vi "XML - Create XML file.vi"(8 "error in (no error)":errorcluster, 11 "CD Wizard - Internal Data":T1) -> (0 "error out":errorcluster, 3 "XML file path":path)   [LabVIEW 2015]
doc: "Create the XML file and alter the content of the file, so that it fits for the generated custom device."
uses:
  TypDef/CD Wizard - Internal data.ctl
  TypDef/CD Wizard - Execution Mode.ctl
  TypDef/CD Wizard - Extra Page Name and GUID.ctl
  TypDef/Create XML-file - States.ctl
  Constants/Constants TypDef/XML File.ctl
  Constants/Constants TypDef/CD System Explorer lvlib.ctl
  TypDef/Target Type.ctl
  Constants/XML File.vi
  Constants/CD System Explorer lvlib.vi
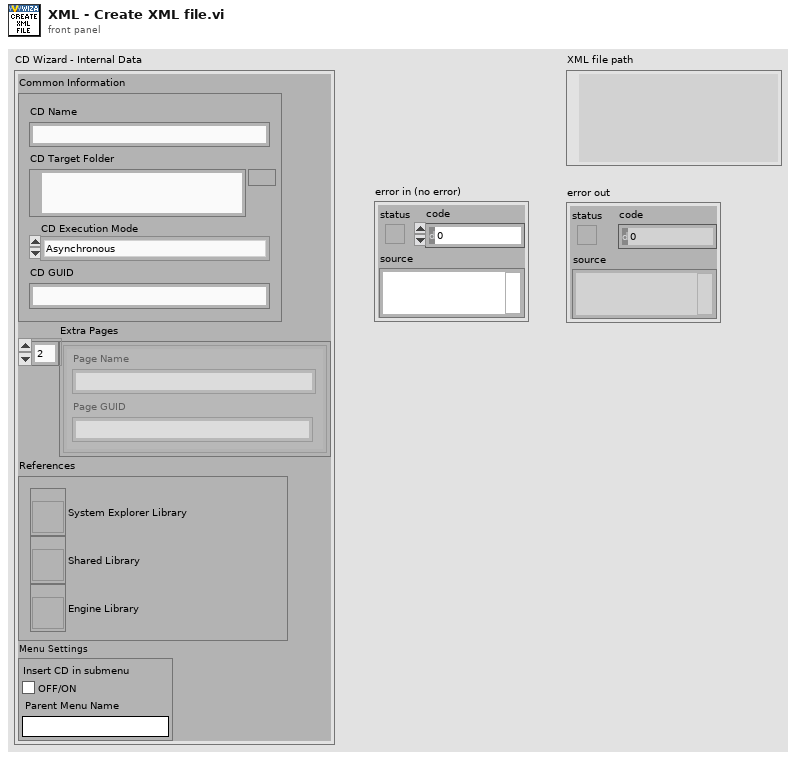
[diagram p1: front panel]
types:
  T1 = typedef "CD Wizard - Internal data.ctl" = cluster{"Common Information":cluster{"CD Name":string, "CD Target Folder":path, "CD Execution Mode":T2, "CD GUID":string}, "Extra Pages":T3[], "References":cluster{"System Explorer Library":refnum<vi>, "Shared Library":refnum<vi>, "Engine Library":refnum<vi>}, "Menu Settings":cluster{"Insert CD in submenu":bool, "Parent Menu Name":string}}
  T2 = typedef "CD Wizard - Execution Mode.ctl" = enum16{"Asynchronous", "Inline HW Interface", "Inline Model Interface", "Inline Timing and Sync", "Asynchronous Timing and Sync"}
  T3 = typedef "CD Wizard - Extra Page Name and GUID.ctl" = cluster{"Page Name":string, "Page GUID":string}
  T4 = typedef "Create XML-file - States.ctl" = enum16{"Initialize", "Copy XML template file", "Read XML file content", "Change CD -MenuName-", "Change CD -Name-", "Change CD -Type-", "Change CD -MainPageGUID-", "Change CD -InitVIPath-", "Change CD -WindowsCustomDeviceVIPath-", "Change CD -WindowsCustomDeviceVIRTPath-", "Change CD -PharlapCustomDeviceVIPath-", "Change CD -PharlapCustomDeviceVIRTPath-", "Change CD -VxWorksCustomDeviceVIPath-", "Change CD -VxWorksCustomDeviceVIRTPath-", "Change CD -LinuxARMCustomDeviceVIPath-", "Change CD -LinuxARMCustomDeviceVIRTPath-", "Change CD -Linuxx64CustomDeviceVIPath-", "Change CD -Linuxx64CustomDeviceVIRTPath-", "Change CD -MainPageVIPath-", "Change CD -ExtraPages-", "Write XML file content back", "Shutdown"}
  T5 = typedef "XML File.ctl" = enum16{"XMLTemplateFilePathAndName", "XMLTimingAndSyncFileName", "XMLCustomDeviceFileName"}
  T6 = typedef "CD System Explorer lvlib.ctl" = enum16{"LibraryFileName", "LibraryFolderName", "System Explorer.FolderName", "System Explorer.Dynamically Called.FolderName", "System Explorer.Dynamically Called.Extra Pages.FolderName", "System Explorer.Dynamically Called.Extra Pages.TemplatePathAndName", "System Explorer.Dynamically Called.Main Page.VIName", "System Explorer.Dynamically Called.Main Page.TemplatePathAndName", "System Explorer.Dynamically Called.Initialization VI.VIName", "System Explorer.Dynamically Called.Initialization VI.TemplatePathAndName", "System Explorer.SubVI.FolderName", "System Explorer.Types.FolderName"}
  T7 = typedef "Target Type.ctl" = enum16{"Windows", "VxWorks", "Pharlap", "Linux 32 ARM", "Linux x64"}
  T8 = enum16{"open", "replace", "create", "open or create", "replace or create", "replace or create with confirmation"}
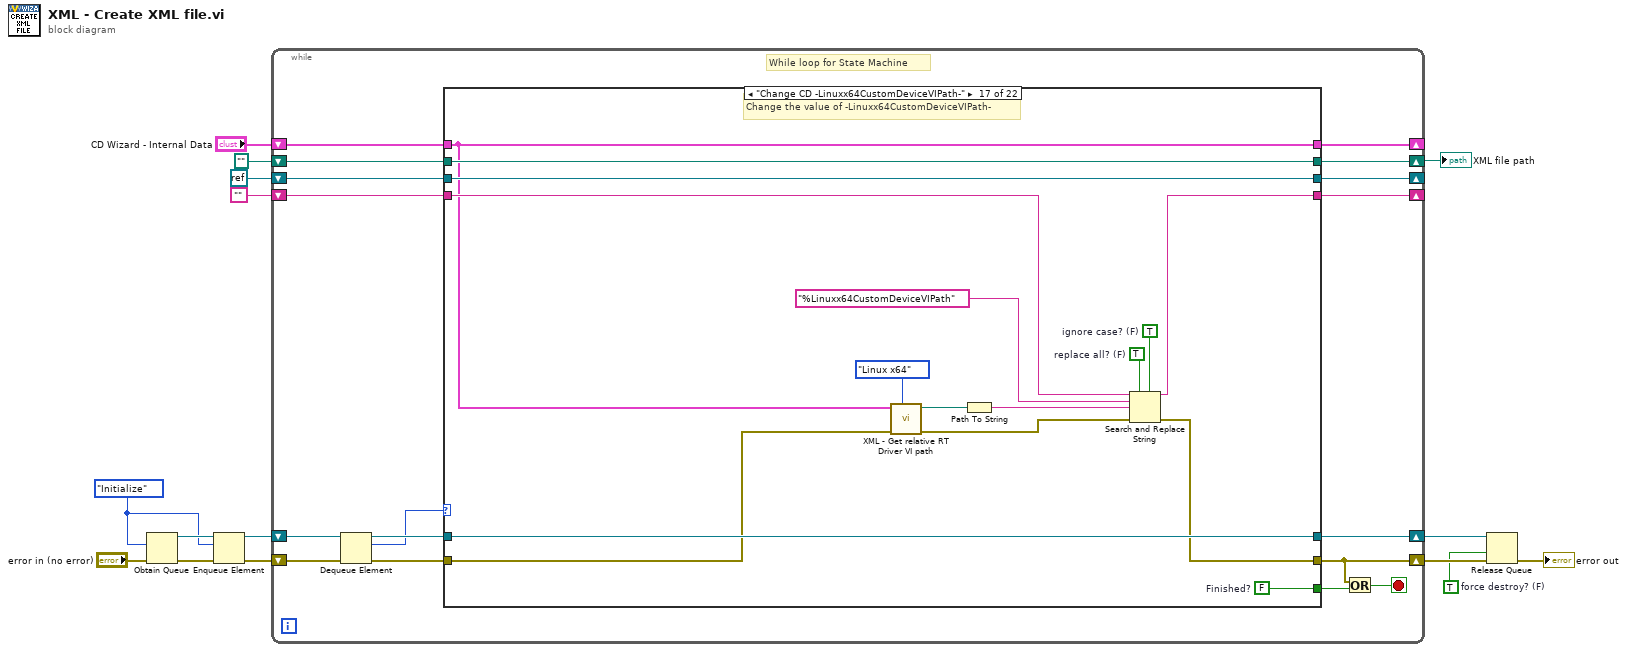
[diagram p0: block diagram]
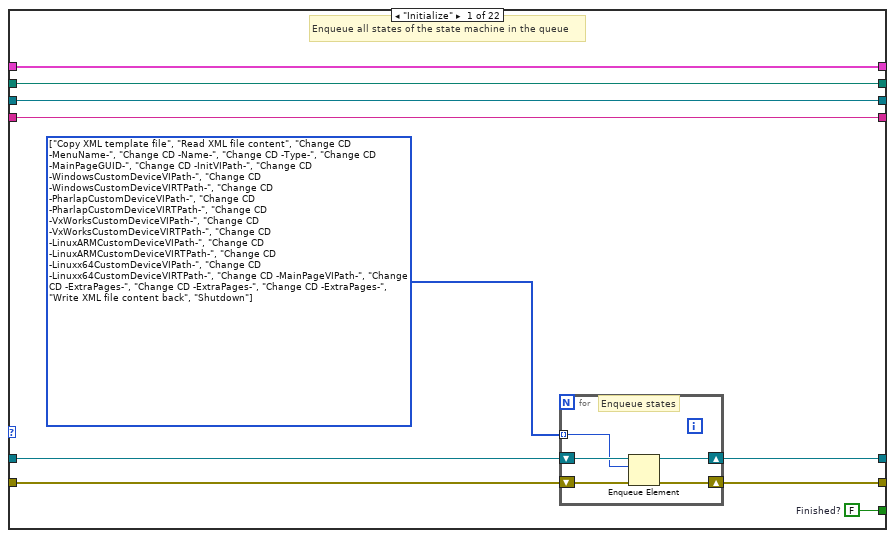
[diagram p2: hidden frame]
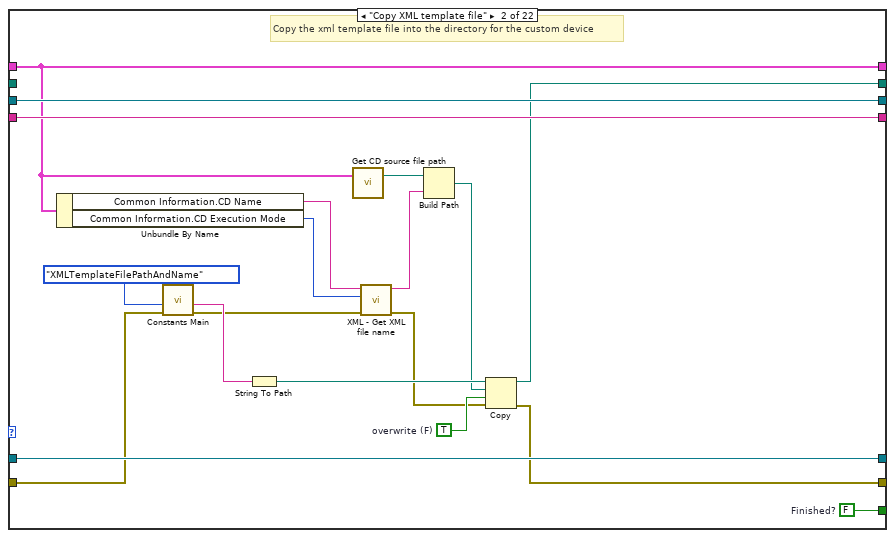
[diagram p3: hidden frame]
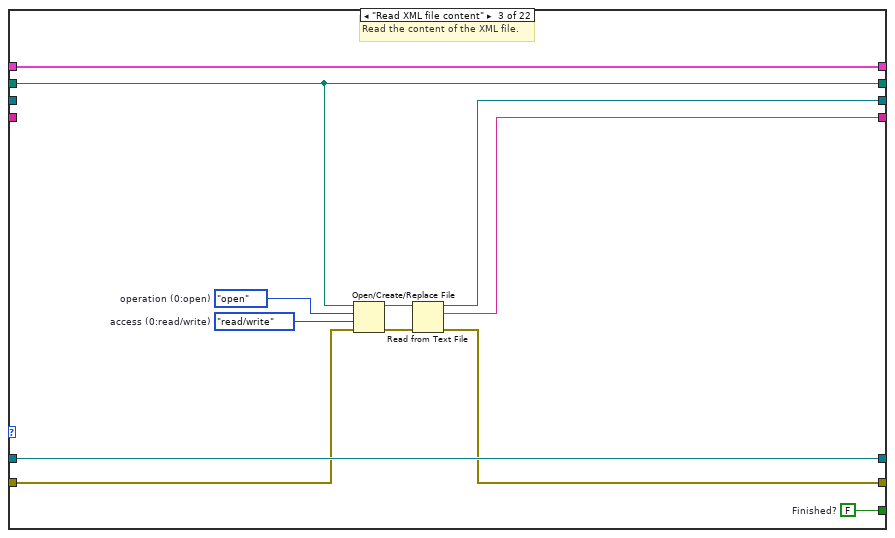
[diagram p4: hidden frame]
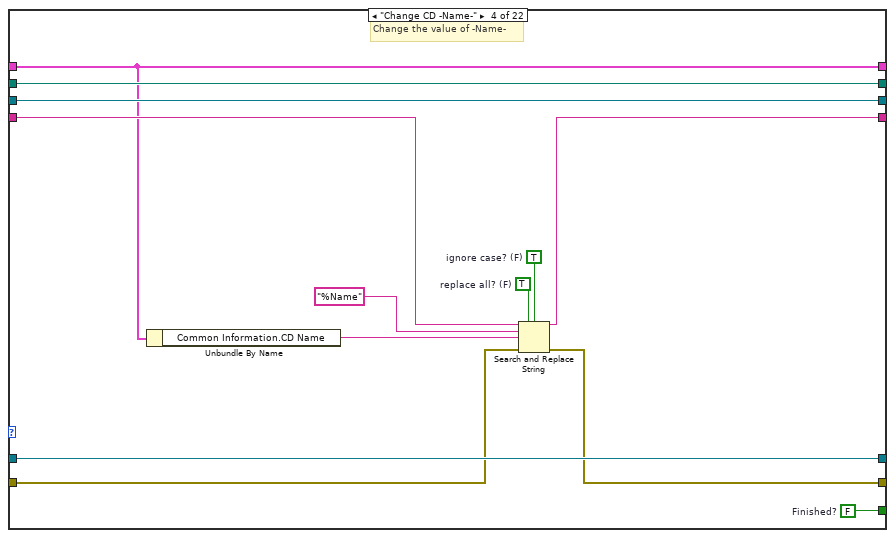
[diagram p5: hidden frame]
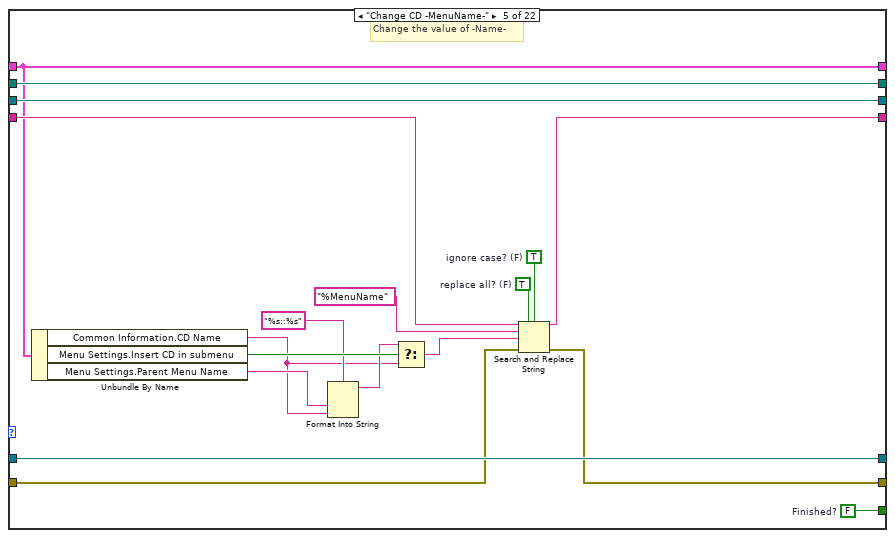
[diagram p6: hidden frame]
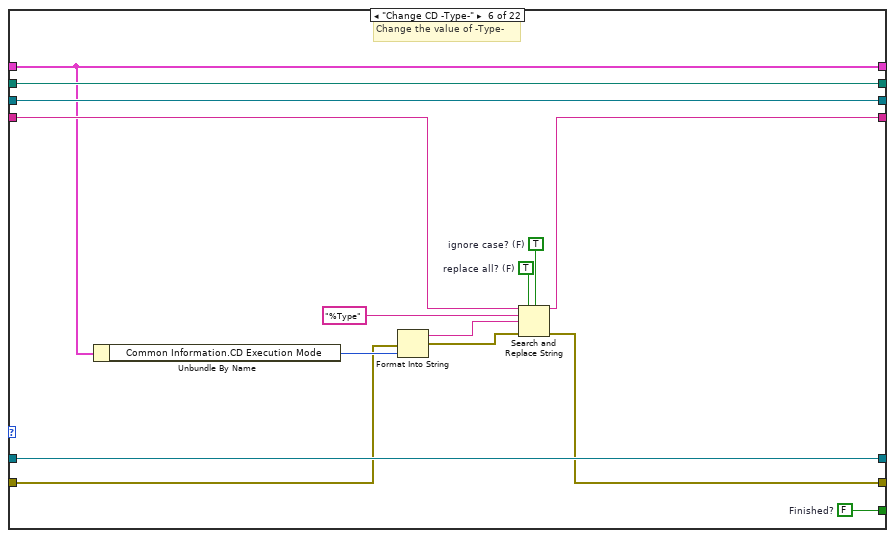
[diagram p7: hidden frame]
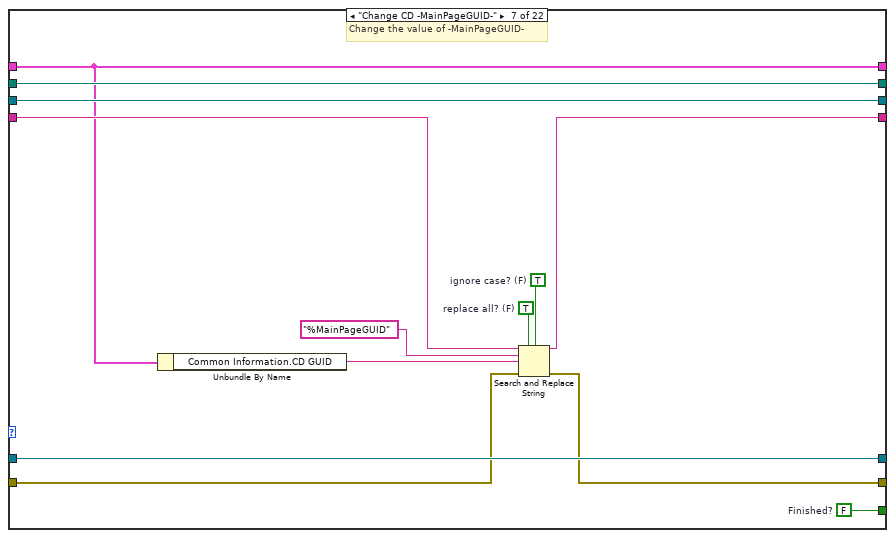
[diagram p8: hidden frame]
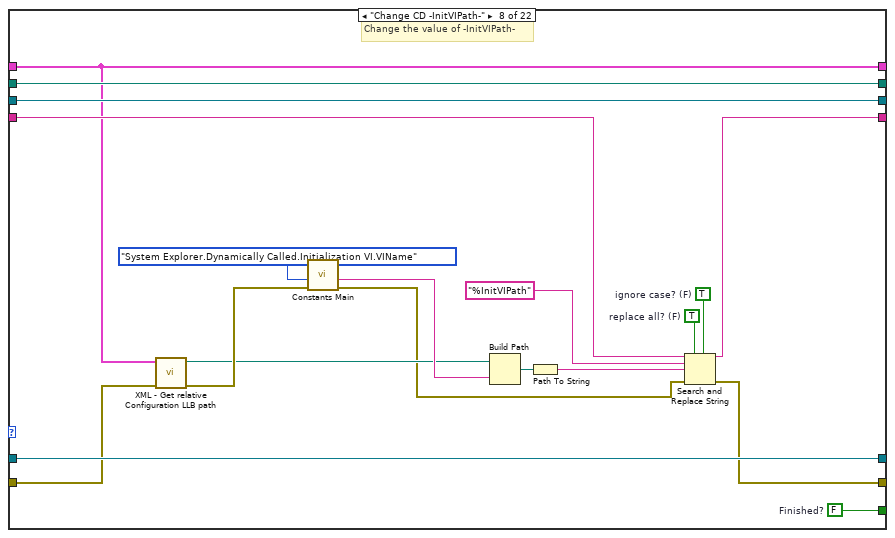
[diagram p9: hidden frame]
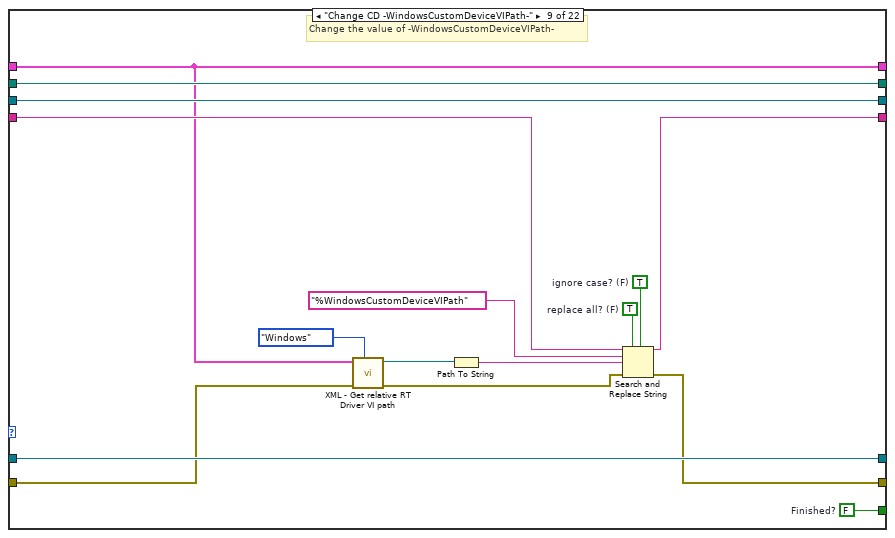
[diagram p10: hidden frame]
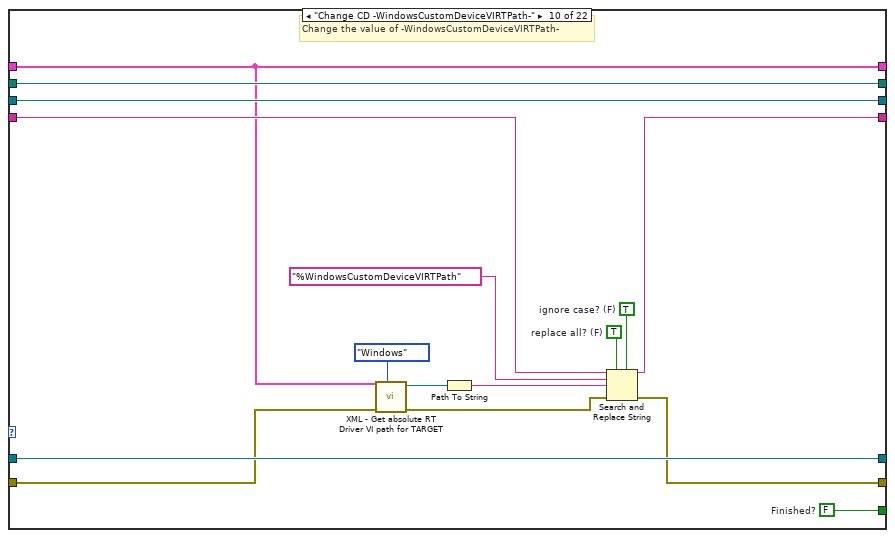
[diagram p11: hidden frame]
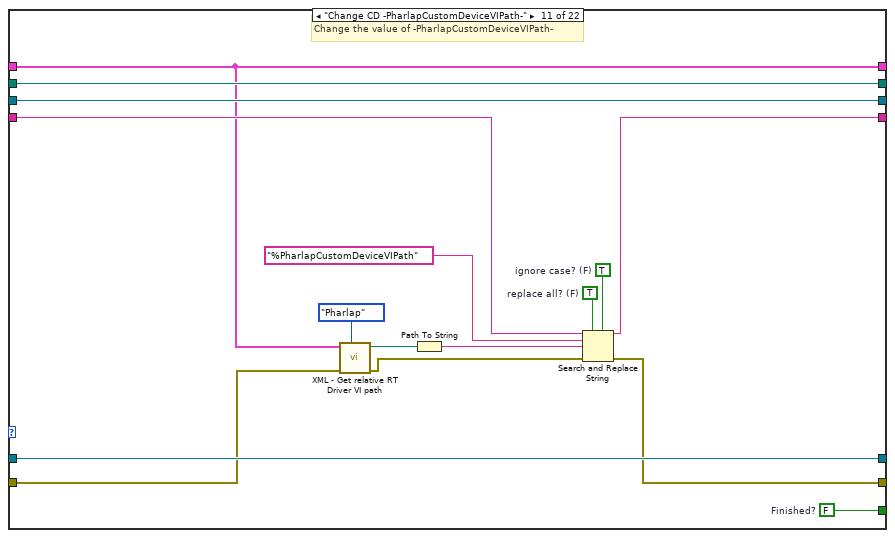
[diagram p12: hidden frame]
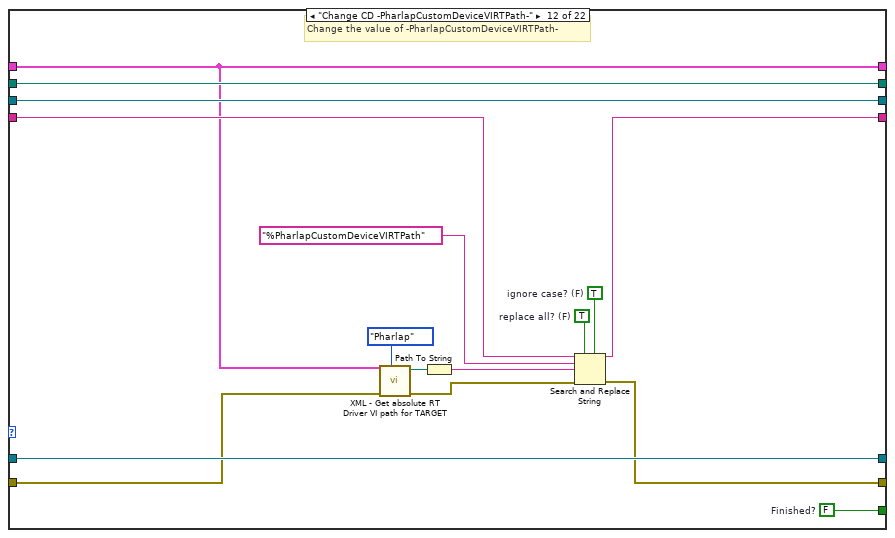
[diagram p13: hidden frame]
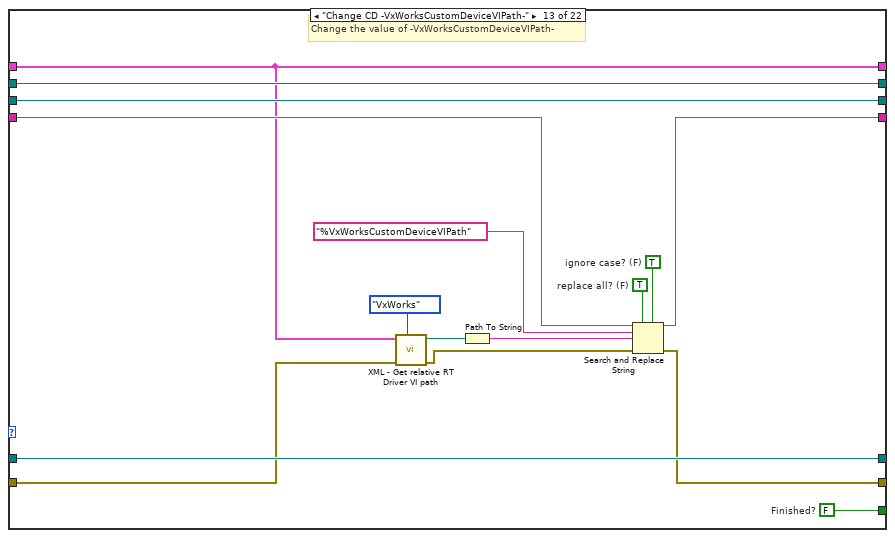
[diagram p14: hidden frame]
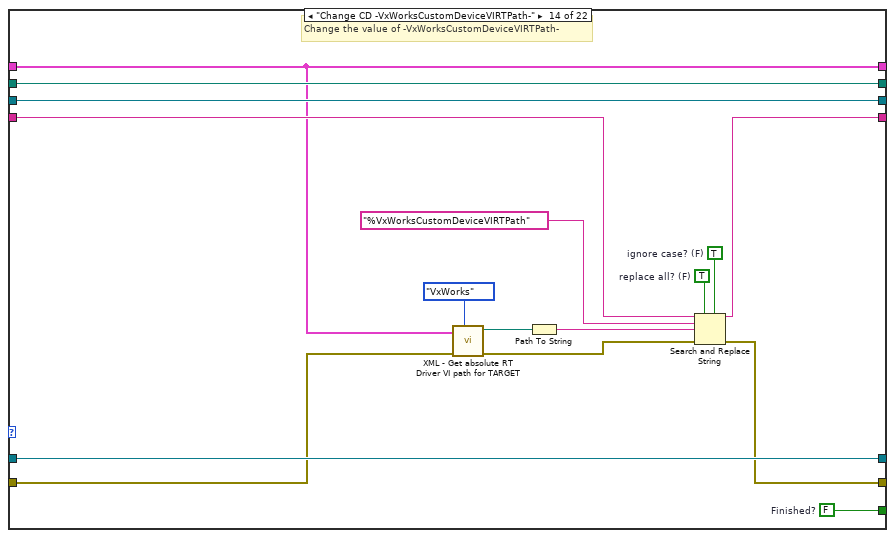
[diagram p15: hidden frame]
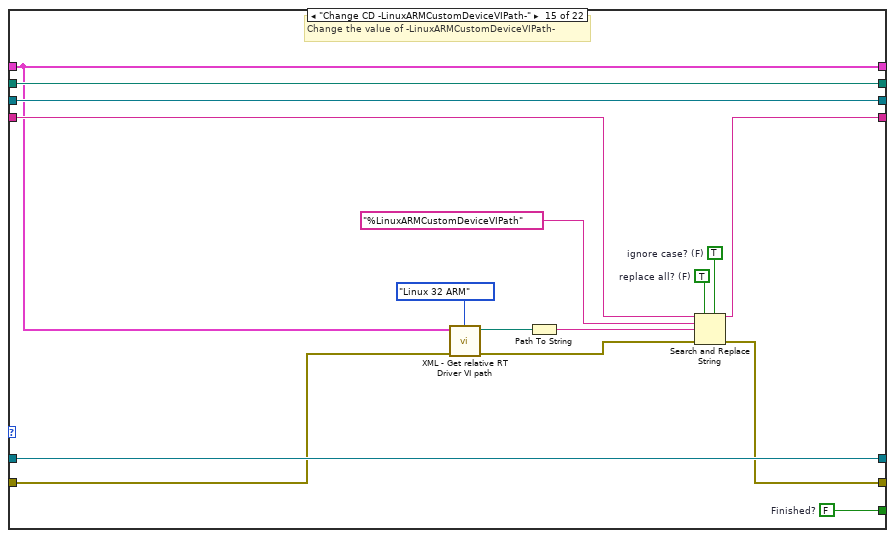
[diagram p16: hidden frame]
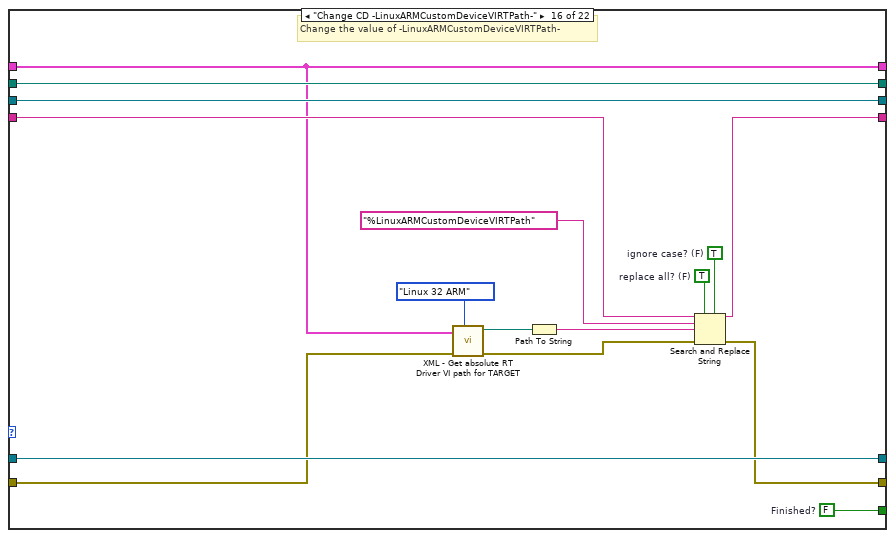
[diagram p17: hidden frame]
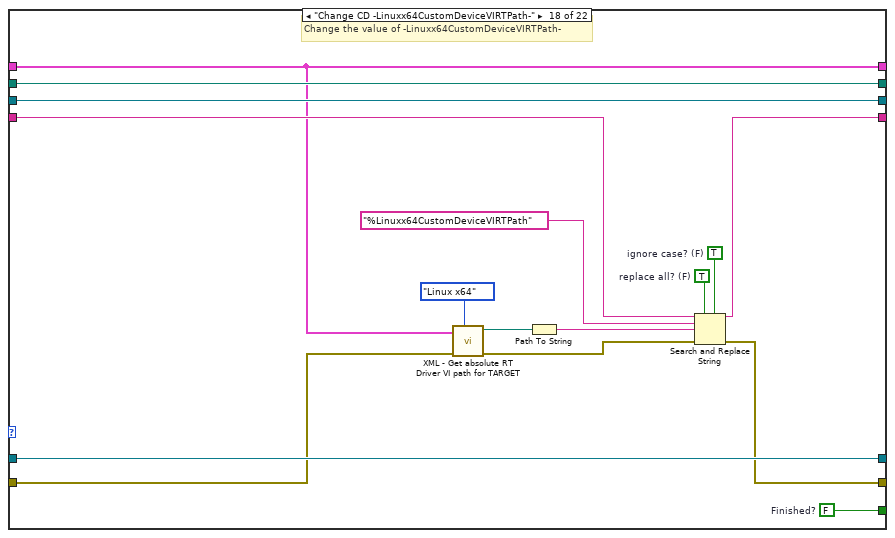
[diagram p18: hidden frame]
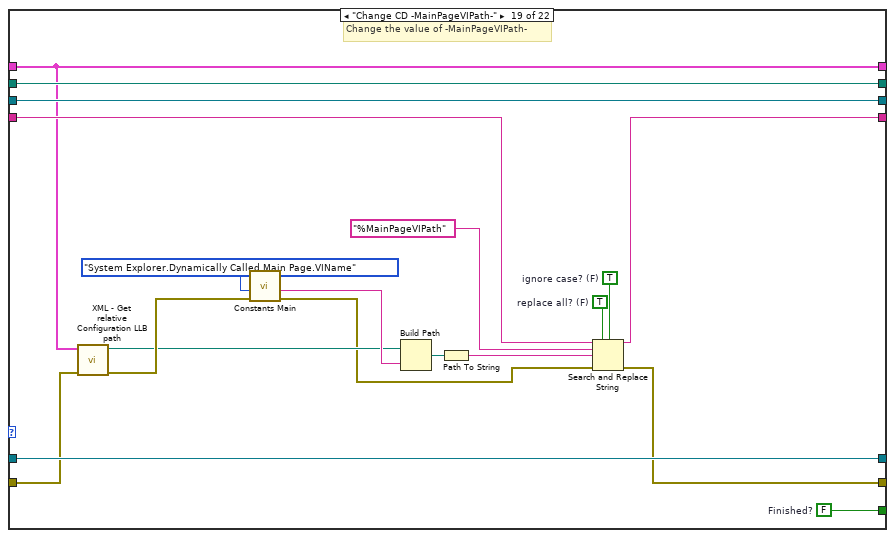
[diagram p19: hidden frame]
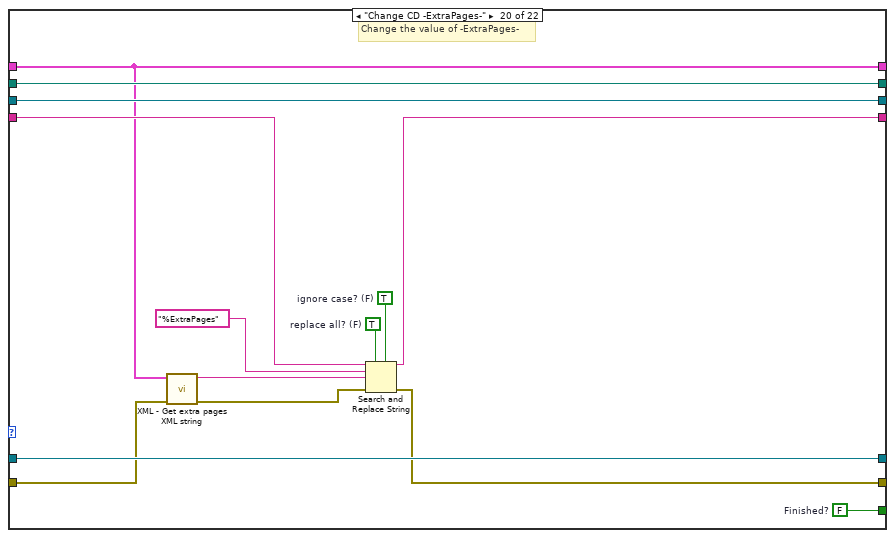
[diagram p20: hidden frame]
diagram:
  w8 = TRUE  # force destroy? (F)
  w5 = Create_XML-file_-_States."Initialize"
  n1 = Obtain Queue(element data type=w5, error in (no error)="error in (no error)") -> (queue out=w14:refnum<queue>, error out=w15:errorcluster)  [unwired: 3 in, 1 out]
  n2 = Enqueue Element(queue=w14, element=w5, error in (no error)=w15) -> (queue out=w13:refnum<queue>, error out=w12:errorcluster)  [unwired: 1 in, 1 out]
  n3 = while {
    shift-right: [w17] -> w9
    shift-left: w12 -> [w31]
    shift-right: [w26] -> _
    shift-left: "CD Wizard - Internal Data" -> [w27]
    shift-right: [w24] -> w1
    shift-left: path "" -> [w23]
    shift-right: [w22] -> _
    shift-left: refnum<k0> refnum -> [w21]
    shift-right: [w19] -> _
    shift-left: "" -> [w20]
    shift-right: [w25] -> w10
    shift-left: w13 -> [w32]
    stop <- w18 stop-if-true
    # "While loop for State Machine"
    n4 = Dequeue Element(queue=w32, error in (no error)=w31) -> (queue out=w29:refnum<queue>, element=w28:T4, error out=w30:errorcluster)  [unwired: 1 in, 1 out]
    n5 = case shown="\"Change CD -Linuxx64CustomDeviceVIPath-\"" w28 {
      tunnel: w30 -> [w35 w59 w73 w84 w102 w112 w127 w146 w159 w177 w191 w206 w223 w239 w255 w271 w287 w303 w318 w336 w355 w374]
      tunnel: w29 -> [w34 w64 w77 w91 w109 w124 w137 w156 w172 w188 w204 w220 w236 w252 w268 w284 w300 w316 w335 w349 w366 w372]
      tunnel: [w36 w58 w71 w85 w103 w118 w131 w150 w168 w183 w199 w215 w231 w247 w263 w279 w295 w311 w329 w343 w354 w374] -> w17
      tunnel: w27 -> [w42 w48 w78 w83 w101 w117 w130 w145 w162 w176 w192 w208 w224 w240 w256 w272 w288 w304 w317 w341 w367 w373]
      tunnel: [w42 w48 w78 w83 w101 w117 w130 w145 w162 w176 w192 w208 w224 w240 w256 w272 w288 w304 w317 w341 w367 w373] -> w26
      tunnel: [w37 w64 w77 w91 w109 w124 w137 w156 w172 w188 w204 w220 w236 w252 w268 w284 w300 w316 w335 w349 w366 w372] -> w25
      tunnel: [w41 w57 w74 w90 w108 w123 w136 w155 w171 w187 w203 w219 w235 w251 w267 w283 w299 w315 w334 w348 w365 w371] -> w24
      tunnel: w23 -> [w41 _ w74 w90 w108 w123 w136 w155 w171 w187 w203 w219 w235 w251 w267 w283 w299 w315 w334 w348 w365 w371]
      tunnel: [w40 w66 w72 w89 w107 w122 w135 w154 w170 w186 w202 w218 w234 w250 w266 w282 w298 w314 w333 w347 w350 w370] -> w22
      tunnel: w21 -> [w40 w66 _ w89 w107 w122 w135 w154 w170 w186 w202 w218 w234 w250 w266 w282 w298 w314 w333 w347 w357 w370]
      tunnel: w20 -> [w39 w65 _ w87 w105 w120 w133 w152 w164 w185 w201 w217 w233 w249 w265 w281 w297 w313 w331 w345 w356 w369]
      tunnel: [w39 w65 w70 w86 w104 w119 w132 w151 w169 w184 w200 w216 w232 w248 w264 w280 w296 w312 w330 w344 w356 w369] -> w19
      tunnel: [w38 w55 w69 w80 w99 w111 w126 w148 w166 w181 w197 w213 w229 w245 w261 w277 w293 w309 w327 w339 w353 w368] -> w16
      frame "Initialize" {
        w33 = T4[] [enum."Copy XML template file", enum."Read XML file content", enum."Change CD -MenuName-", enum."Change CD -Name-", enum."Change CD -Type-", enum."Change CD -MainPageGUID-", enum."Change CD -InitVIPath-", enum."Change CD -WindowsCustomDeviceVIPath-", enum."Change CD -WindowsCustomDeviceVIRTPath-", enum."Change CD -PharlapCustomDeviceVIPath-", enum."Change CD -PharlapCustomDeviceVIRTPath-", enum."Change CD -VxWorksCustomDeviceVIPath-", enum."Change CD -VxWorksCustomDeviceVIRTPath-", enum."Change CD -LinuxARMCustomDeviceVIPath-", enum."Change CD -LinuxARMCustomDeviceVIRTPath-", enum."Change CD -Linuxx64CustomDeviceVIPath-", enum."Change CD -Linuxx64CustomDeviceVIRTPath-", enum."Change CD -MainPageVIPath-", enum."Change CD -ExtraPages-", enum."Change CD -ExtraPages-", enum."Change CD -ExtraPages-", enum."Write XML file content back", enum."Shutdown"] items=["Initialize", "Copy XML template file", "Read XML file content", "Change CD -MenuName-", "Change CD -Name-", "Change CD -Type-", "Change CD -MainPageGUID-", "Change CD -InitVIPath-", "Change CD -WindowsCustomDeviceVIPath-", "Change CD -WindowsCustomDeviceVIRTPath-", "Change CD -PharlapCustomDeviceVIPath-", "Change CD -PharlapCustomDeviceVIRTPath-", "Change CD -VxWorksCustomDeviceVIPath-", "Change CD -VxWorksCustomDeviceVIRTPath-", "Change CD -LinuxARMCustomDeviceVIPath-", "Change CD -LinuxARMCustomDeviceVIRTPath-", "Change CD -Linuxx64CustomDeviceVIPath-", "Change CD -Linuxx64CustomDeviceVIRTPath-", "Change CD -MainPageVIPath-", "Change CD -ExtraPages-", "Write XML file content back", "Shutdown"]
        w38 = FALSE  # Finished?
        # "Enqueue all states of the state machine in the queue"
        n6 = for {
          shift-right: [w46] -> w37
          shift-left: w34 -> [w47]
          shift-right: [w45] -> w36
          shift-left: w35 -> [w44]
          tunnel: w33 -> [w43] mode=indexing
          # "Enqueue states"
          n7 = Enqueue Element(queue=w47, element=w43, error in (no error)=w44) -> (queue out=w46:refnum<queue>, error out=w45:errorcluster)  [unwired: 1 in, 1 out]
        }
      }
      frame "Copy XML template file" {
        w55 = FALSE  # Finished?
        w56 = TRUE  # overwrite (F)
        # "Copy the xml template file into the directory for the custom device"
        n8 = Unbundle By Name(w48) -> ("Common Information.CD Name"=w54:string, "Common Information.CD Execution Mode"=w53:T2)
        n9 = call-poly "Constants Main.vi"("error in (no error)"=w59, "Action"=XML_File."XMLTemplateFilePathAndName") -> ("error out"=w51:errorcluster, "Output"=w62:string)  [unwired: 8 in]
        n10 = String To Path(string=w62) -> (path=w61:path)
        n11 = call "Get CD source file path.vi"("CD Wizard - Internal Data"=w48) -> ("CD Source file path"=w49:path)  [unwired: 2 in]
        n12 = call "XML - Get XML file name.vi"("error in (no error)"=w51, "CD Execution Mode (Asynchronous)"=w53, "CD Name"=w54) -> ("error out"=w50:errorcluster, "XML file name"=w52:string)  [unwired: 7 in]
        n13 = Build Path(base path=w49, name or relative path=w52) -> (appended path=w60:path)
        n14 = Copy(8:w50, 9:w56, 10:w60, 11:w61) -> (0:w58:errorcluster, 3:w57:path)  [unwired: 2 out]
      }
      frame "Read XML file content" {
        w67 = T8."open"  # operation (0:open)
        w68 = enum16{"read/write", "read-only", "write-only"}."read/write"  # access (0:read/write)
        w69 = FALSE  # Finished?
        # "Read the content of the XML file."
        n15 = Open/Create/Replace File(file path (use dialog)=w74, error in=w73, operation (0:open)=w67, access (0:read/write)=w68) -> (refnum out=w76:refnum<file>, error out=w75:errorcluster)  [unwired: 3 out]
        n16 = Read from Text File(file (use dialog)=w76, error in=w75) -> (refnum out=w72:refnum<file>, text=w70:string, error out=w71:errorcluster)  [unwired: 3 out]
      }
      frame "Change CD -Name-" {
        w79 = TRUE  # ignore case? (F)
        w80 = FALSE  # Finished?
        w81 = TRUE  # replace all? (F)
        # "Change the value of -Name-"
        n17 = Unbundle By Name(w83) -> ("Common Information.CD Name"=w82:string)
        n18 = Search and Replace String(replace all?=w81, case sensitive?=w79, input string=w87, search string="%Name", replace string=w82, error in=w84) -> (result string=w86:string, error out=w85:errorcluster)  [unwired: 1 in, 3 out]
      }
      frame "Change CD -MenuName-" {
        w98 = TRUE  # ignore case? (F)
        w99 = FALSE  # Finished?
        w100 = TRUE  # replace all? (F)
        # "Change the value of -Name-"
        n19 = Unbundle By Name(w101) -> ("Common Information.CD Name"=w93:string, "Menu Settings.Insert CD in submenu"=w97:bool, "Menu Settings.Parent Menu Name"=w95:string)
        n20 = Format Into String(format string="%s::%s", w95, w93) -> (resulting string=w94:string)  [unwired: 2 in, 1 out]
        n21 = Select(t=w94, s=w97, f=w93) -> (s? t:f=w92:string)
        n22 = Search and Replace String(replace all?=w100, case sensitive?=w98, input string=w105, search string="%MenuName", replace string=w92, error in=w102) -> (result string=w104:string, error out=w103:errorcluster)  [unwired: 1 in, 3 out]
      }
      frame "Change CD -Type-" {
        w110 = TRUE  # ignore case? (F)
        w111 = FALSE  # Finished?
        w116 = TRUE  # replace all? (F)
        # "Change the value of -Type-"
        n23 = Unbundle By Name(w117) -> ("Common Information.CD Execution Mode"=w115:T2)
        n24 = Format Into String(error in=w112, w115) -> (resulting string=w114:string, error out=w113:errorcluster)  [unwired: 2 in]
        n25 = Search and Replace String(replace all?=w116, case sensitive?=w110, input string=w120, search string="%Type", replace string=w114, error in=w113) -> (result string=w119:string, error out=w118:errorcluster)  [unwired: 1 in, 3 out]
      }
      frame "Change CD -MainPageGUID-" {
        w125 = TRUE  # ignore case? (F)
        w126 = FALSE  # Finished?
        w129 = TRUE  # replace all? (F)
        # "Change the value of -MainPageGUID-"
        n26 = Unbundle By Name(w130) -> ("Common Information.CD GUID"=w128:string)
        n27 = Search and Replace String(replace all?=w129, case sensitive?=w125, input string=w133, search string="%MainPageGUID", replace string=w128, error in=w127) -> (result string=w132:string, error out=w131:errorcluster)  [unwired: 1 in, 3 out]
      }
      frame "Change CD -InitVIPath-" {
        w147 = TRUE  # ignore case? (F)
        w148 = FALSE  # Finished?
        w149 = TRUE  # replace all? (F)
        # "Change the value of -InitVIPath-"
        n28 = call "XML - Get relative Configuration LLB path.vi"("error in (no error)"=w146, "CD Wizard - Internal Data"=w145) -> ("error out"=w140:errorcluster, "Relative Configuration LLB path"=w139:path)  [unwired: 8 in]
        n29 = call-poly "Constants Main.vi"("error in (no error)"=w140, "Action"=CD_System_Explorer_lvlib."System Explorer.Dynamically Called.Initialization VI.VIName") -> ("error out"=w138:errorcluster, "Output"=w143:string)  [unwired: 8 in]
        n30 = Build Path(base path=w139, name or relative path=w143) -> (appended path=w141:path)
        n31 = Path To String(path=w141) -> (string=w144:string)
        n32 = Search and Replace String(replace all?=w149, case sensitive?=w147, input string=w152, search string="%InitVIPath", replace string=w144, error in=w138) -> (result string=w151:string, error out=w150:errorcluster)  [unwired: 1 in, 3 out]
      }
      frame "Change CD -WindowsCustomDeviceVIPath-" {
        w165 = TRUE  # ignore case? (F)
        w166 = FALSE  # Finished?
        w167 = TRUE  # replace all? (F)
        # "Change the value of -WindowsCustomDeviceVIPath-"
        n33 = call "XML - Get relative RT Driver VI path.vi"("Target Type (Windows)"=Target_Type."Windows", "error in (no error)"=w159, "CD Wizard - Internal Data"=w162) -> ("error out"=w157:errorcluster, "Relative RT Driver VI path"=w158:path)  [unwired: 7 in]
        n34 = Path To String(path=w158) -> (string=w161:string)
        n35 = Search and Replace String(replace all?=w167, case sensitive?=w165, input string=w164, search string="%WindowsCustomDeviceVIPath", replace string=w161, error in=w157) -> (result string=w169:string, error out=w168:errorcluster)  [unwired: 1 in, 3 out]
      }
      frame "Change CD -WindowsCustomDeviceVIRTPath-" {
        w180 = TRUE  # ignore case? (F)
        w181 = FALSE  # Finished?
        w182 = TRUE  # replace all? (F)
        # "Change the value of -WindowsCustomDeviceVIRTPath-"
        n36 = call "XML - Get absolute RT Driver VI path for TARGET.vi"("Target Type (Windows)"=Target_Type."Windows", "error in (no error)"=w177, "CD Wizard - Internal Data"=w176) -> ("error out"=w178:errorcluster, "Relative RT Driver TARGET path"=w173:path)  [unwired: 7 in]
        n37 = Path To String(path=w173) -> (string=w175:string)
        n38 = Search and Replace String(replace all?=w182, case sensitive?=w180, input string=w185, search string="%WindowsCustomDeviceVIRTPath", replace string=w175, error in=w178) -> (result string=w184:string, error out=w183:errorcluster)  [unwired: 1 in, 3 out]
      }
      frame "Change CD -PharlapCustomDeviceVIPath-" {
        w196 = TRUE  # ignore case? (F)
        w197 = FALSE  # Finished?
        w198 = TRUE  # replace all? (F)
        # "Change the value of -PharlapCustomDeviceVIPath-"
        n39 = call "XML - Get relative RT Driver VI path.vi"("Target Type (Windows)"=Target_Type."Pharlap", "error in (no error)"=w191, "CD Wizard - Internal Data"=w192) -> ("error out"=w194:errorcluster, "Relative RT Driver VI path"=w189:path)  [unwired: 7 in]
        n40 = Path To String(path=w189) -> (string=w190:string)
        n41 = Search and Replace String(replace all?=w198, case sensitive?=w196, input string=w201, search string="%PharlapCustomDeviceVIPath", replace string=w190, error in=w194) -> (result string=w200:string, error out=w199:errorcluster)  [unwired: 1 in, 3 out]
      }
      frame "Change CD -PharlapCustomDeviceVIRTPath-" {
        w212 = TRUE  # ignore case? (F)
        w213 = FALSE  # Finished?
        w214 = TRUE  # replace all? (F)
        # "Change the value of -PharlapCustomDeviceVIRTPath-"
        n42 = call "XML - Get absolute RT Driver VI path for TARGET.vi"("Target Type (Windows)"=Target_Type."Pharlap", "error in (no error)"=w206, "CD Wizard - Internal Data"=w208) -> ("error out"=w210:errorcluster, "Relative RT Driver TARGET path"=w205:path)  [unwired: 7 in]
        n43 = Path To String(path=w205) -> (string=w207:string)
        n44 = Search and Replace String(replace all?=w214, case sensitive?=w212, input string=w217, search string="%PharlapCustomDeviceVIRTPath", replace string=w207, error in=w210) -> (result string=w216:string, error out=w215:errorcluster)  [unwired: 1 in, 3 out]
      }
      frame "Change CD -VxWorksCustomDeviceVIPath-" {
        w228 = TRUE  # ignore case? (F)
        w229 = FALSE  # Finished?
        w230 = TRUE  # replace all? (F)
        # "Change the value of -VxWorksCustomDeviceVIPath-"
        n45 = call "XML - Get relative RT Driver VI path.vi"("Target Type (Windows)"=Target_Type."VxWorks", "error in (no error)"=w223, "CD Wizard - Internal Data"=w224) -> ("error out"=w226:errorcluster, "Relative RT Driver VI path"=w221:path)  [unwired: 7 in]
        n46 = Path To String(path=w221) -> (string=w222:string)
        n47 = Search and Replace String(replace all?=w230, case sensitive?=w228, input string=w233, search string="%VxWorksCustomDeviceVIPath", replace string=w222, error in=w226) -> (result string=w232:string, error out=w231:errorcluster)  [unwired: 1 in, 3 out]
      }
      frame "Change CD -VxWorksCustomDeviceVIRTPath-" {
        w244 = TRUE  # ignore case? (F)
        w245 = FALSE  # Finished?
        w246 = TRUE  # replace all? (F)
        # "Change the value of -VxWorksCustomDeviceVIRTPath-"
        n48 = call "XML - Get absolute RT Driver VI path for TARGET.vi"("Target Type (Windows)"=Target_Type."VxWorks", "error in (no error)"=w239, "CD Wizard - Internal Data"=w240) -> ("error out"=w242:errorcluster, "Relative RT Driver TARGET path"=w237:path)  [unwired: 7 in]
        n49 = Path To String(path=w237) -> (string=w238:string)
        n50 = Search and Replace String(replace all?=w246, case sensitive?=w244, input string=w249, search string="%VxWorksCustomDeviceVIRTPath", replace string=w238, error in=w242) -> (result string=w248:string, error out=w247:errorcluster)  [unwired: 1 in, 3 out]
      }
      frame "Change CD -LinuxARMCustomDeviceVIPath-" {
        w260 = TRUE  # ignore case? (F)
        w261 = FALSE  # Finished?
        w262 = TRUE  # replace all? (F)
        # "Change the value of -LinuxARMCustomDeviceVIPath-"
        n51 = call "XML - Get relative RT Driver VI path.vi"("Target Type (Windows)"=Target_Type."Linux 32 ARM", "error in (no error)"=w255, "CD Wizard - Internal Data"=w256) -> ("error out"=w253:errorcluster, "Relative RT Driver VI path"=w254:path)  [unwired: 7 in]
        n52 = Path To String(path=w254) -> (string=w258:string)
        n53 = Search and Replace String(replace all?=w262, case sensitive?=w260, input string=w265, search string="%LinuxARMCustomDeviceVIPath", replace string=w258, error in=w253) -> (result string=w264:string, error out=w263:errorcluster)  [unwired: 1 in, 3 out]
      }
      frame "Change CD -LinuxARMCustomDeviceVIRTPath-" {
        w276 = TRUE  # ignore case? (F)
        w277 = FALSE  # Finished?
        w278 = TRUE  # replace all? (F)
        # "Change the value of -LinuxARMCustomDeviceVIRTPath-"
        n54 = call "XML - Get absolute RT Driver VI path for TARGET.vi"("Target Type (Windows)"=Target_Type."Linux 32 ARM", "error in (no error)"=w271, "CD Wizard - Internal Data"=w272) -> ("error out"=w274:errorcluster, "Relative RT Driver TARGET path"=w269:path)  [unwired: 7 in]
        n55 = Path To String(path=w269) -> (string=w270:string)
        n56 = Search and Replace String(replace all?=w278, case sensitive?=w276, input string=w281, search string="%LinuxARMCustomDeviceVIRTPath", replace string=w270, error in=w274) -> (result string=w280:string, error out=w279:errorcluster)  [unwired: 1 in, 3 out]
      }
      frame "Change CD -Linuxx64CustomDeviceVIPath-" {
        w292 = TRUE  # ignore case? (F)
        w293 = FALSE  # Finished?
        w294 = TRUE  # replace all? (F)
        # "Change the value of -Linuxx64CustomDeviceVIPath-"
        n57 = call "XML - Get relative RT Driver VI path.vi"("Target Type (Windows)"=Target_Type."Linux x64", "error in (no error)"=w287, "CD Wizard - Internal Data"=w288) -> ("error out"=w285:errorcluster, "Relative RT Driver VI path"=w286:path)  [unwired: 7 in]
        n58 = Path To String(path=w286) -> (string=w290:string)
        n59 = Search and Replace String(replace all?=w294, case sensitive?=w292, input string=w297, search string="%Linuxx64CustomDeviceVIPath", replace string=w290, error in=w285) -> (result string=w296:string, error out=w295:errorcluster)  [unwired: 1 in, 3 out]
      }
      frame "Change CD -Linuxx64CustomDeviceVIRTPath-" {
        w308 = TRUE  # ignore case? (F)
        w309 = FALSE  # Finished?
        w310 = TRUE  # replace all? (F)
        # "Change the value of -Linuxx64CustomDeviceVIRTPath-"
        n60 = call "XML - Get absolute RT Driver VI path for TARGET.vi"("Target Type (Windows)"=Target_Type."Linux x64", "error in (no error)"=w303, "CD Wizard - Internal Data"=w304) -> ("error out"=w306:errorcluster, "Relative RT Driver TARGET path"=w301:path)  [unwired: 7 in]
        n61 = Path To String(path=w301) -> (string=w302:string)
        n62 = Search and Replace String(replace all?=w310, case sensitive?=w308, input string=w313, search string="%Linuxx64CustomDeviceVIRTPath", replace string=w302, error in=w306) -> (result string=w312:string, error out=w311:errorcluster)  [unwired: 1 in, 3 out]
      }
      frame "Change CD -MainPageVIPath-" {
        w326 = TRUE  # ignore case? (F)
        w327 = FALSE  # Finished?
        w328 = TRUE  # replace all? (F)
        # "Change the value of -MainPageVIPath-"
        n63 = call "XML - Get relative Configuration LLB path.vi"("error in (no error)"=w318, "CD Wizard - Internal Data"=w317) -> ("error out"=w322:errorcluster, "Relative Configuration LLB path"=w321:path)  [unwired: 8 in]
        n64 = call-poly "Constants Main.vi"("error in (no error)"=w322, "Action"=CD_System_Explorer_lvlib."System Explorer.Dynamically Called.Main Page.VIName") -> ("error out"=w319:errorcluster, "Output"=w325:string)  [unwired: 8 in]
        n65 = Build Path(base path=w321, name or relative path=w325) -> (appended path=w323:path)
        n66 = Path To String(path=w323) -> (string=w320:string)
        n67 = Search and Replace String(replace all?=w328, case sensitive?=w326, input string=w331, search string="%MainPageVIPath", replace string=w320, error in=w319) -> (result string=w330:string, error out=w329:errorcluster)  [unwired: 1 in, 3 out]
      }
      frame "Change CD -ExtraPages-" {
        w338 = TRUE  # ignore case? (F)
        w339 = FALSE  # Finished?
        w342 = TRUE  # replace all? (F)
        # "Change the value of -ExtraPages-"
        n68 = call "XML - Get extra pages XML string.vi"("error in (no error)"=w336, "CD Wizard - Internal Data"=w341) -> ("error out"=w337:errorcluster, "Extra Pages XML string"=w340:string)  [unwired: 8 in]
        n69 = Search and Replace String(replace all?=w342, case sensitive?=w338, input string=w345, search string="%ExtraPages", replace string=w340, error in=w337) -> (result string=w344:string, error out=w343:errorcluster)  [unwired: 1 in, 3 out]
      }
      frame "Write XML file content back" {
        w350 = refnum<file> refnum  # refnum out
        w353 = FALSE  # Finished?
        w358 = enum16{"start", "end", "current"}."start"  # from (0:start)
        # "Write the modified file content back to the XML file"
        n70 = String Length(string=w356) -> (length=w352:i32)
        n71 = Set File Position(refnum=w357, from (0:start)=w358, error in=w355) -> (refnum out=w359:refnum<file>, error out=w360:errorcluster)  [unwired: 1 out]
        n72 = To Quad Integer(1:w352) -> (0:w351:i64)
        n73 = Set File Size(4:w360, 6:w351, 7:w359) -> (0:w362:errorcluster, 3:w361:refnum<file>)
        n74 = Write to Text File(file (use dialog)=w361, text=w356, error in=w362) -> (refnum out=w364:refnum<file>, error out=w363:errorcluster)  [unwired: 2 out]
        n75 = Close File(refnum=w364, error in=w363) -> (error out=w354:errorcluster)  [unwired: 1 out]
      }
      frame "Shutdown" {
        w368 = TRUE  # Finished?
        # "Shut down the state machine"
      }
    }
    n76 = Or(x=w17, y=w16) -> (x .or. y?=w18:bool)
  }
  "XML file path" <- w1
  n77 = Release Queue(queue=w10, force destroy? (F)=w8, error in (no error)=w9) -> (error out=→"error out":errorcluster)  [unwired: 2 out]
